vi "Get Device Properties List.vi"(0 "SLSC Local in":refnum<class "SLSC Local.lvclass">, 11 "error in (no error)":errorcluster) -> (4 "SLSC Local out":refnum<class "SLSC Local.lvclass">, 8 "Sys.DeviceProperties":refnum<k21>[](array[refnum]), 15 "error out":errorcluster)   [LabVIEW 2015, in "SLSC Local.lvclass"]
uses:
  SLSC Local.lvclass
  <resource>/objmgr/slsc.rc
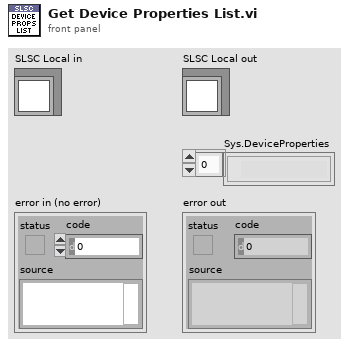
[diagram p1: front panel]
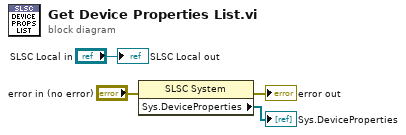
[diagram p0: block diagram]
diagram:
  n1 = property class="SLSC System"(error in="error in (no error)") -> (error out=→"error out":errorcluster, "Sys.DeviceProperties"=→"Sys.DeviceProperties":refnum<k21>[])  [unwired: 1 in, 1 out]
  "SLSC Local out" <- "SLSC Local in"
